vi "Get Phasor Configuration.vi"(8 "error in (no error)":errorcluster, 9 "Phasor Index":i32, 10 "PMU Index":i32, 11 "Pseudo PDC ID":i32) -> (0 "error out":errorcluster, 2 "Phasor Name":string, 3 "Phasor Configuration":T1)   [LabVIEW 2017, in "PMU Recorder Light.lvlib" / "Statnett C37.118 DLL.lvclass"]
uses:
  Statnett C37.118 DLL.lvclass
  c37118-dll/C37118-DLL.lvlib
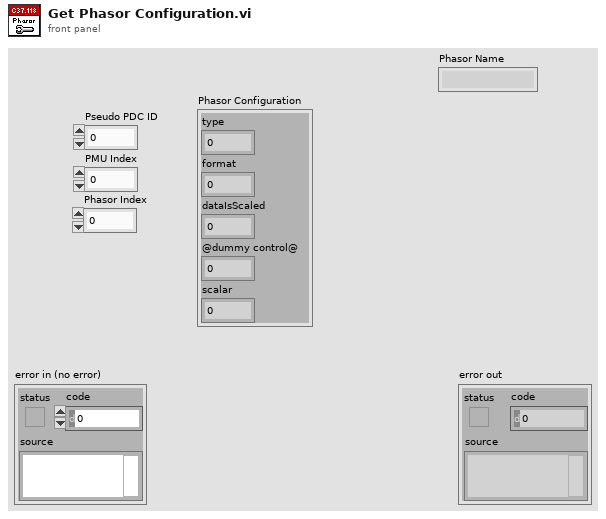
[diagram p1: front panel]
types:
  T1 = cluster{"type":u8, "format":u8, "dataIsScaled":u8, "@dummy control@":i8, "scalar":sgl}
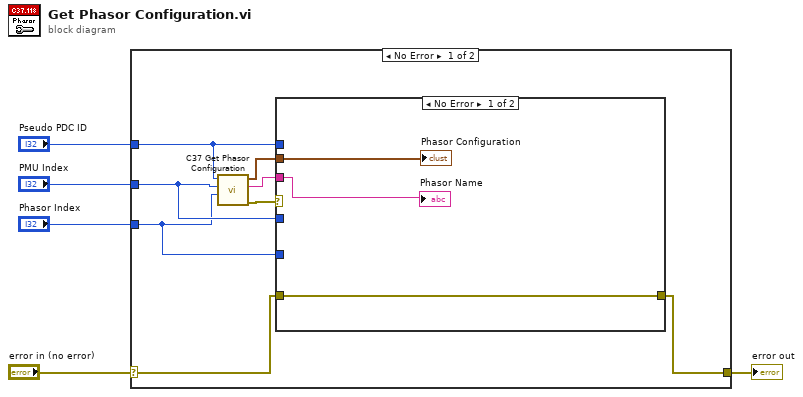
[diagram p0: block diagram]
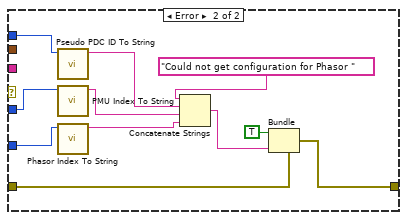
[diagram p2: hidden frame]
diagram:
  n1 = case shown="No Error" "error in (no error)" {
    selector: "error in (no error)" -> [w13 w28]
    tunnel: [w12 w28] -> w4
    tunnel: "Pseudo PDC ID" -> [w11 _]
    tunnel: "PMU Index" -> [w10 _]
    tunnel: "Phasor Index" -> [w9 _]
    frame No Error {
      n2 = call "C37 Get Phasor Configuration.vi"("Phasor Index"=w9, "PMU Index"=w10, "Pseudo PDC ID"=w11) -> ("error out"=w8:errorcluster, "Channel Name"=w6:string, "Phasor Configuration"=w7:T1)  [unwired: 6 in]
      n3 = case shown="No Error" w8 {
        tunnel: w13 -> [w16 w27]
        tunnel: w10 -> [_ w20]
        tunnel: [w16 w23] -> w12
        tunnel: w7 -> [w15 _]
        tunnel: w6 -> [w14 _]
        tunnel: w11 -> [_ w22]
        tunnel: w9 -> [_ w21]
        frame No Error {
          "Phasor Name" <- w14
          "Phasor Configuration" <- w15
        }
        frame Error {
          n4 = call "Pseudo PDC ID To String.vi"("Pseudo PDC ID"=w22) -> ("String"=w19:string)  [unwired: 10 in]
          n5 = call "PMU Index To String.vi"("PMU Index"=w20) -> ("String"=w18:string)  [unwired: 10 in]
          n6 = call "Phasor Index To String.vi"("Phasor Index"=w21) -> ("String"=w17:string)  [unwired: 10 in]
          n7 = Concatenate Strings("Could not get configuration for Phasor " ("source"), w19, w18, w17) -> (w24:string)
          n8 = Bundle(cluster=w27, "status"=TRUE, "source"=w24) -> (w23:errorcluster)  [unwired: 1 in]
        }
      }
    }
    frame Error {
    }
  }
  "error out" <- w4
